vi "Table.vi"(4 "Cellspacing (0)":i32, 5 "Cellpadding (0)":i32, 6 "Class (\"\")":string, 8 "Array of Rows (Empty Array)":string[](array[string]), 9 "Previous HTML in":string) -> (3 "HTML out":string)   [LabVIEW 2011]
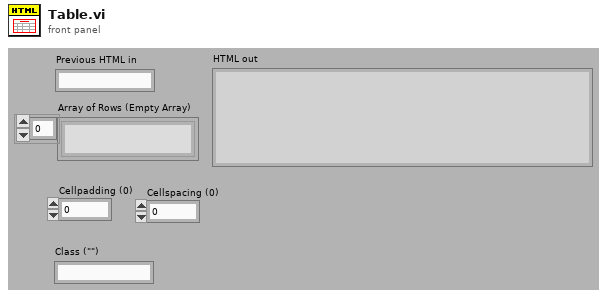
[diagram p1: front panel]
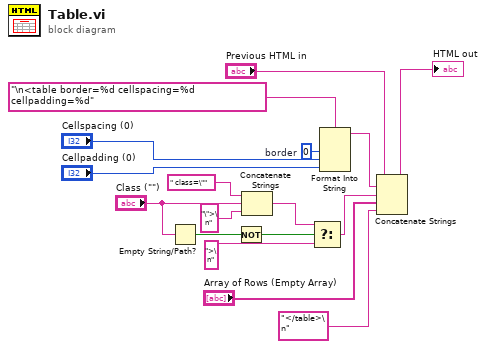
[diagram p0: block diagram]
diagram:
  w5 = 0  # border
  n1 = Empty String/Path?(string/path="Class (\"\")") -> (empty?=w14:bool)
  n2 = Not(x=w14) -> (.not. x?=w8:bool)
  n3 = Concatenate Strings(" class=\"", "Class (\"\")", "\">\n") -> (w10:string)
  n4 = Select(t=w10, s=w8, f=">\n") -> (s? t:f=w2:string)
  n5 = Format Into String(format string="\n<table border=%d cellspacing=%d cellpadding=%d", w5, "Cellspacing (0)", "Cellpadding (0)") -> (resulting string=w6:string)  [unwired: 2 in, 1 out]
  n6 = Concatenate Strings("Previous HTML in", w6, w2, "Array of Rows (Empty Array)", "</table>\n") -> (→"HTML out":string)
